vi "Set wpsel ready.vi"(8 "error in (no error)":errorcluster, 11 "ICS in":refnum<class "ICS.lvclass">) -> (0 "error out":errorcluster, 3 "ICS out":refnum<class "ICS.lvclass">)   [LabVIEW 2018, in "ICS.lvclass"]
uses:
  ICS.lvclass
  Motor/Motor.lvclass
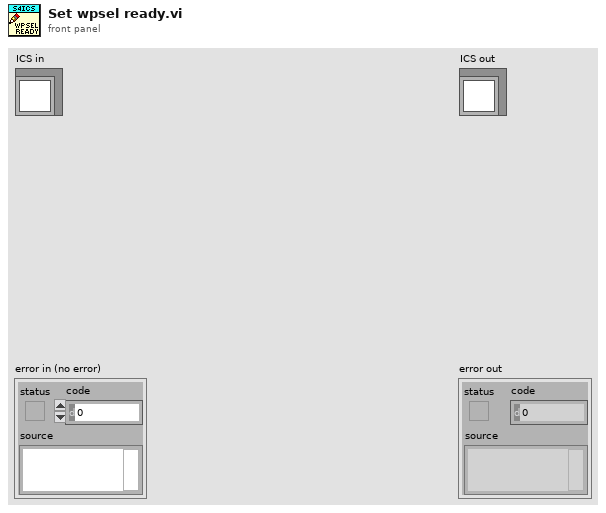
[diagram p1: front panel]
types:
  T1 = cluster{"mode":string, "condition":string, "position":string, "pos_name":string, "pos_id":string}
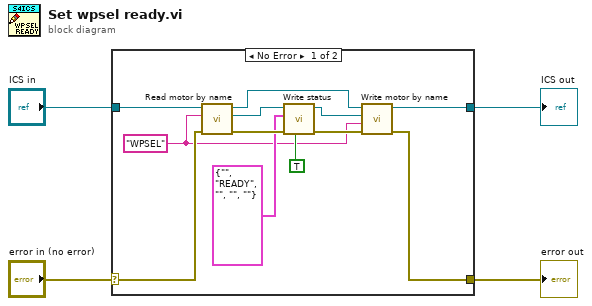
[diagram p0: block diagram]
diagram:
  n1 = case shown="No Error" "error in (no error)" {
    selector: "error in (no error)" -> [w15 w17]
    tunnel: [w9 w17] -> w3
    tunnel: [w8 w18] -> w1
    tunnel: "ICS in" -> [w16 w18]
    frame No Error {
      w5 = "WPSEL" ("motor name")
      n2 = call-dynamic "Read motor by name.vi"("error in (no error)"=w15, "motor name"=w5, "ICS in"=w16) -> ("error out"=w13:errorcluster, "Motor.lvclass"=w12:refnum<class "Motor.lvclass">, "ICS out"=w7:refnum<class "ICS.lvclass">)  [unwired: 5 in, 1 out]
      n3 = call-dynamic "Write status.vi"("hold if empty"=TRUE, "error in (no error)"=w13, "status"=T1 {"mode"="", "condition"="READY", "position"="", "pos_name"="", "pos_id"=""}, "Motor in"=w12) -> ("error out"=w10:errorcluster, "Motor out"=w6:refnum<class "Motor.lvclass">)  [unwired: 6 in]
      n4 = call-dynamic "Write motor by name.vi"("error in (no error)"=w10, "name"=w5, "motor"=w6, "ICS in"=w7) -> ("error out"=w9:errorcluster, "ICS out"=w8:refnum<class "ICS.lvclass">)  [unwired: 6 in]
    }
    frame Error {
    }
  }
  "error out" <- w3
  "ICS out" <- w1
